vi "Change sign.vi"(9 "Boolean":bool, 10 "y":dbl, 11 "x":dbl) -> (2 "-y":dbl, 3 "-x":dbl)   [LabVIEW 2012]
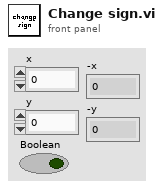
[diagram p1: front panel]
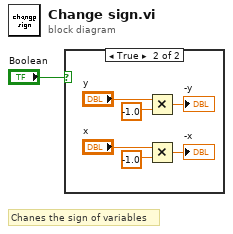
[diagram p0: block diagram]
diagram:
  # "Chanes the sign of variables"
  n1 = case shown="True" "Boolean" {
    frame False {
    }
    frame True {
      n2 = Multiply(x="y", y=-1.0) -> (x*y=→"-y":dbl)
      n3 = Multiply(x="x", y=-1.0) -> (x*y=→"-x":dbl)
    }
  }
